vi "Scratch.vi"() -> ()   [LabVIEW 2026]
panel:
  in  "stop":bool
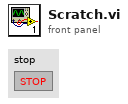
[diagram p1: front panel]
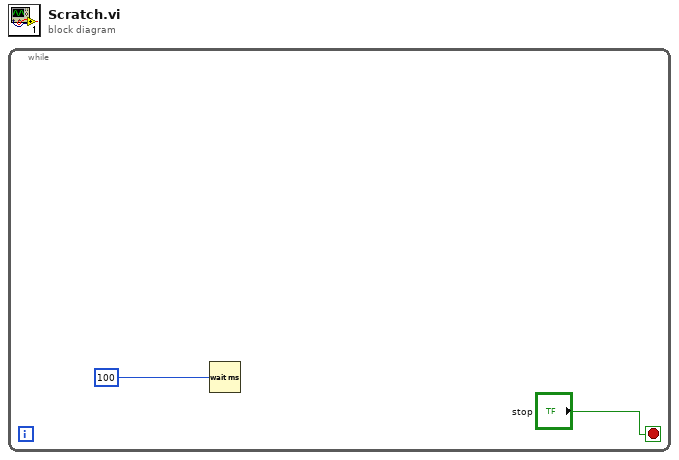
[diagram p0: block diagram]
diagram:
  n1 = while {
    stop <- "stop" stop-if-true
    n2 = Wait (ms)(milliseconds to wait=i16 100) -> ()  [unwired: 1 out]
  }
